vi "SEK 2019.vi"() -> ()   [LabVIEW 2016]
uses:
  <vilib>/NXT/Subs/LVHSConnector.ctl
  <vilib>/NXT/LegoClasses/BrickReference/BrickReference.lvclass
  <vilib>/NXT/Block Support/NXT_InputPort.ctl
  <vilib>/NXT/Block Support/NXT_OutputPort.ctl
  <vilib>/NXT/Dual Mode Library/Sensors/EV3_Ultrasonic_CM.vi
  <vilib>/NXT/NXTIO Xnodes/NXTIONodeSubVIs/NXTStopMotors.vi
  <vilib>/NXT/Dual Mode Library/Sensors/EV3_Color_Reflect.vi
  <vilib>/NXT/NXTIO Xnodes/NXTIONodeSubVIs/NXTMoveMotors.vi
  <vilib>/NXT/NXTIO Xnodes/AddressXNode/NXTIOAddress.xnode
  <vilib>/NXT/NXTIO Xnodes/NXTIOXNode/NXTIO.xnode
panel:
  in  "Preto EV3 (menor que y)":sgl
  in  "Branco EV3 (maior que x)":sgl=17.0
  in  "Port Ultra Topo":T1=2 items=["Port 1", "Port 2", "Port 3", "Port 4"]
  in  "Port Color Left":T1 items=["Port 1", "Port 2", "Port 3", "Port 4"]
  in  "Port Color Right":T1 items=["Port 1", "Port 2", "Port 3", "Port 4"]
  in  "Amarelo HiTechnic":i32=6
  in  "Azul HiTechnic":i32=3
  in  "Vermelho HiTechnic":i32=8
  in  "Chão (cm)":sgl=20.0
  in  "Verde HiTechnic":i32=6
  in  "Preto HiTechnic":i32
  in  "Port Gyro":T1 items=["Port 1", "Port 2", "Port 3", "Port 4"]
  in  "Port Ultra Base":T1=2 items=["Port 1", "Port 2", "Port 3", "Port 4"]
  in  "Port Color HiTechnic":T1=1 items=["Port 1", "Port 2", "Port 3", "Port 4"]
  in  "Branco HiTechnic":i32=17
  in  "NXT/EV3":T2
  # "PARÂMETROS HITECHNIC"
  # "PARÂMETROS ULTRASSOM"
  # "PORTAS DE SENSORES"
  # "PARÂMETROS COR"
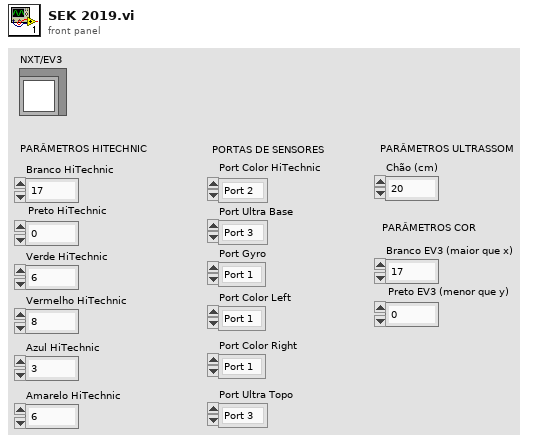
[diagram p1: front panel]
types:
  T1 = typedef "NXT_InputPort.ctl" = u32
  T2 = typedef "LVHSConnector.ctl" = refnum<class "BrickReference.lvclass">
  T3 = cluster{"Color Number":i32, "Red":i32, "Green":i32, "Blue":i32, "White Level":i32}
  T4 = typedef "NXT_OutputPort.ctl" = u8
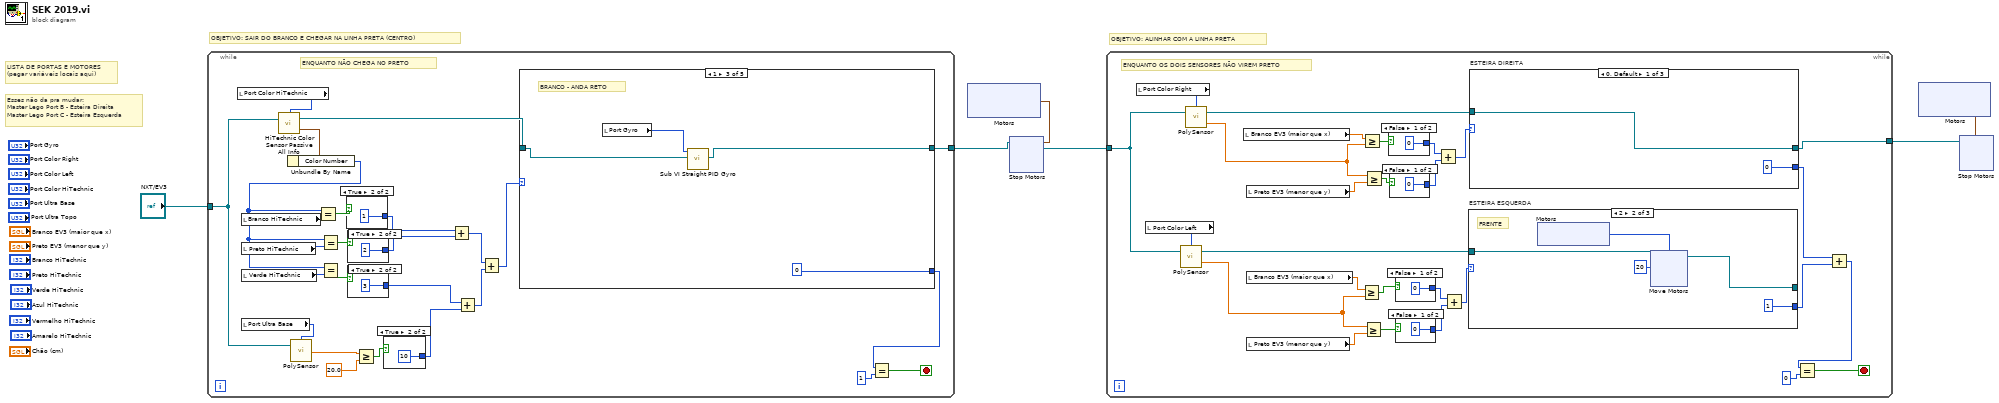
[diagram p0: block diagram]
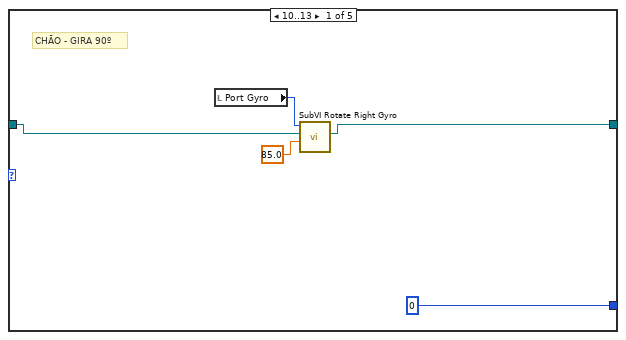
[diagram p2: hidden frame]
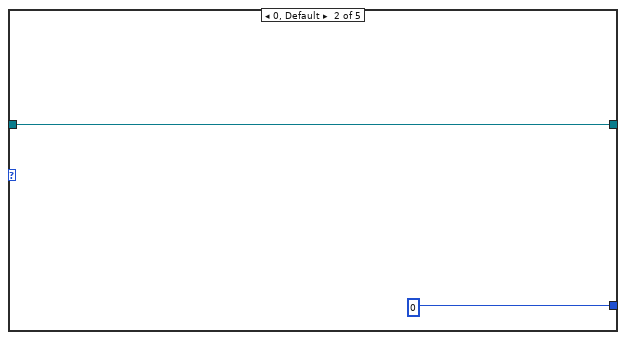
[diagram p3: hidden frame]
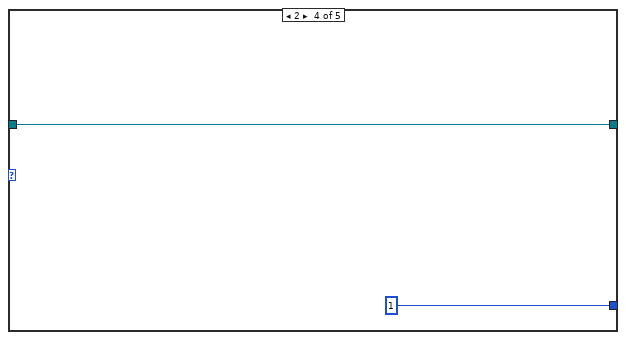
[diagram p4: hidden frame]
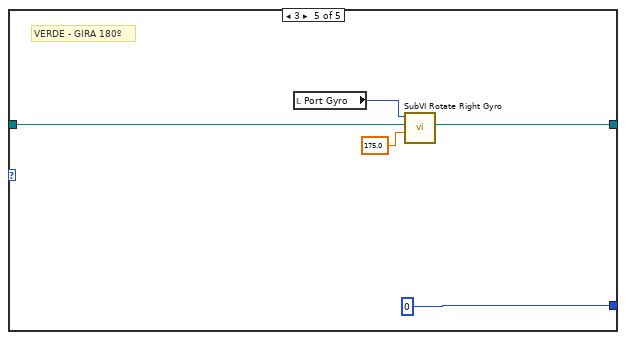
[diagram p5: hidden frame]
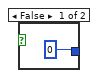
[diagram p6: hidden frame]
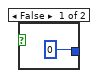
[diagram p7: hidden frame]
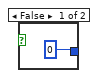
[diagram p8: hidden frame]
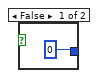
[diagram p9: hidden frame]
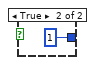
[diagram p10: hidden frame]
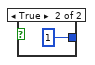
[diagram p11: hidden frame]
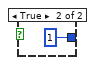
[diagram p12: hidden frame]
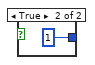
[diagram p13: hidden frame]
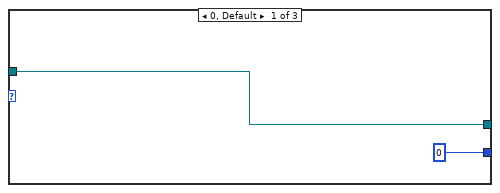
[diagram p14: hidden frame]
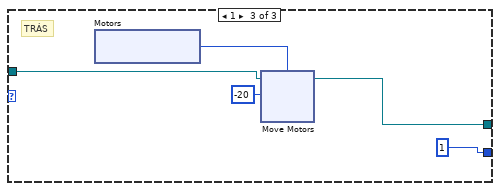
[diagram p15: hidden frame]
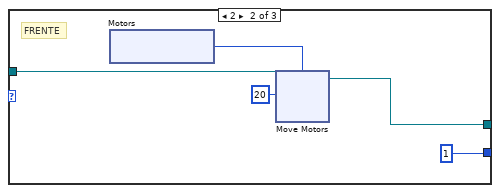
[diagram p16: hidden frame]
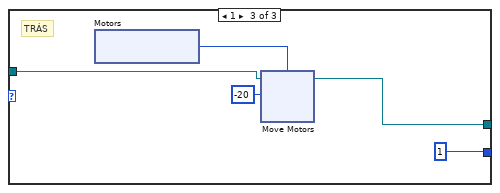
[diagram p17: hidden frame]
diagram:
  # "OBJETIVO: ALINHAR COM A LINHA PRETA"
  # "LISTA DE PORTAS E MOTORES\n(pegar variáveis locais aqui)"
  # "Esses não da pra mudar:\nMaster Lego Port B - Esteira Direita\nMaster Lego Port C - Esteira Esquerda"
  # "OBJETIVO: SAIR DO BRANCO E CHEGAR NA LINHA PRETA (CENTRO)"
  n1 = while {
    tunnel: "NXT/EV3" -> [w12]
    tunnel: [w7] -> w1
    stop <- w27 stop-if-true
    # "ENQUANTO NÃO CHEGA NO PRETO"
    n2 = local read "Port Color HiTechnic"() -> (w14:T1)
    n3 = local read "Branco HiTechnic"() -> (w25:i32)
    n4 = local read "Port Ultra Base"() -> (w9:T1)
    n5 = local read "Preto HiTechnic"() -> (w8:i32)
    n6 = local read "Verde HiTechnic"() -> (w26:i32)
    n7 = call <vilib>:"HiTechnic Color Sensor Passive All Info.vi"("NXT"=w12, "Port"=w14) -> ("All Info"=w11:T3, "NXT"=w13:T2)  [unwired: 1 in]
    n8 = Unbundle By Name(w11) -> ("Color Number"=w10:i32)
    n9 = call-poly <vilib>:"PolySensor.vi"("NXT/EV3"=w12, "Port (Port 1)"=w9) -> ("Centimeters"=w16:sgl)  [unwired: 1 in, 1 out]
    n10 = Equal?(x=w10, y=w25) -> (x = y?=w32:bool)
    n11 = Equal?(x=w10, y=w8) -> (x = y?=w31:bool)
    n12 = Equal?(x=w10, y=w26) -> (x = y?=w30:bool)
    n13 = case shown="True" w32 {
      tunnel: [0 1] -> w24
      frame False {
      }
      frame True {
      }
    }
    n14 = case shown="True" w31 {
      tunnel: [0 2] -> w23
      frame False {
      }
      frame True {
      }
    }
    n15 = case shown="True" w30 {
      tunnel: [0 3] -> w22
      frame False {
      }
      frame True {
      }
    }
    n16 = Greater Or Equal?(x=w16, y=sgl 20.0) -> (x >= y?=w17:bool)
    n17 = case shown="True" w17 {
      tunnel: [0 10] -> w21
      frame False {
      }
      frame True {
      }
    }
    n18 = Add(x=w24, y=w23) -> (x+y=w20:i32)
    n19 = Add(x=w22, y=w21) -> (x+y=w19:i32)
    n20 = Add(x=w20, y=w19) -> (x+y=w18:i32)
    n21 = case shown="1" w18 {
      tunnel: w13 -> [w35 w39 w42 w44 w49]
      tunnel: [w34 w39 w41 w44 w47] -> w7
      tunnel: [0 0 0 1 0] -> w28
      frame 10..13 {
        # "CHÃO - GIRA 90º"
        n22 = local read "Port Gyro"() -> (w33:T1)
        n23 = call "SubVI Rotate Right Gyro.vi"("angle"=85.0 ("Degrees"), "NXT/EV3"=w35, "PortGyro"=w33) -> ("NXT/EV3 2"=w34:T2)  [unwired: 7 in]
      }
      frame 0, Default {
      }
      frame 1 {
        # "BRANCO - ANDA RETO"
        n24 = local read "Port Gyro"() -> (w40:T1)
        n25 = call "Sub VI Straight PID Gyro.vi"("NXT/EV3"=w42, "PortGyro"=w40) -> ("NXT/EV3 2"=w41:T2)  [unwired: 9 in]
      }
      frame 2 {
      }
      frame 3 {
        # "VERDE - GIRA 180º"
        n26 = local read "Port Gyro"() -> (w46:T1)
        n27 = call "SubVI Rotate Right Gyro.vi"("angle"=175.0 ("Degrees"), "NXT/EV3"=w49, "PortGyro"=w46) -> ("NXT/EV3 2"=w47:T2)  [unwired: 7 in]
      }
    }
    n28 = Equal?(x=w28, y=1) -> (x = y?=w27:bool)
  }
  n29 = xnode "Motors"() -> ("Motor"=w5:cluster{"Port":T4, "Port":T4})
  n30 = xnode "Stop Motors"("Motors"=w5, "NXT/EV3"=w1) -> ("NXT/EV3"=w4:T2)
  n31 = while {
    tunnel: w4 -> [w85]
    tunnel: [w64] -> w2
    stop <- w62 stop-if-true
    # "ENQUANTO OS DOIS SENSORES NÃO VIREM PRETO"
    n32 = local read "Port Color Right"() -> (w84:T1)
    n33 = local read "Port Color Left"() -> (w83:T1)
    n34 = call-poly <vilib>:"PolySensor.vi"("NXT/EV3"=w85, "Port (Port 1)"=w83) -> ("Scaled Value"=w75:sgl, "NXT/EV3"=w81:T2)  [unwired: 1 in]
    n35 = call-poly <vilib>:"PolySensor.vi"("NXT/EV3"=w85, "Port (Port 1)"=w84) -> ("Scaled Value"=w76:sgl, "NXT/EV3"=w82:T2)  [unwired: 1 in]
    n36 = local read "Branco EV3 (maior que x)"() -> (w80:sgl)
    n37 = local read "Preto EV3 (menor que y)"() -> (w79:sgl)
    n38 = local read "Branco EV3 (maior que x)"() -> (w78:sgl)
    n39 = local read "Preto EV3 (menor que y)"() -> (w77:sgl)
    n40 = Greater Or Equal?(x=w78, y=w75) -> (x >= y?=w67:bool)
    n41 = Greater Or Equal?(x=w80, y=w76) -> (x >= y?=w74:bool)
    n42 = Greater Or Equal?(x=w75, y=w77) -> (x >= y?=w66:bool)
    n43 = Greater Or Equal?(x=w76, y=w79) -> (x >= y?=w73:bool)
    n44 = case shown="False" w74 {
      tunnel: [0 1] -> w71
      frame False {
      }
      frame True {
      }
    }
    n45 = case shown="False" w73 {
      tunnel: [0 1] -> w70
      frame False {
      }
      frame True {
      }
    }
    n46 = case shown="False" w67 {
      tunnel: [0 1] -> w69
      frame False {
      }
      frame True {
      }
    }
    n47 = case shown="False" w66 {
      tunnel: [0 1] -> w68
      frame False {
      }
      frame True {
      }
    }
    n48 = Add(x=w71, y=w70) -> (x+y=w72:i32)
    n49 = Add(x=w69, y=w68) -> (x+y=w65:i32)
    n50 = case "ESTEIRA ESQUERDA" shown="2" w65 {
      tunnel: w81 -> [w95 w99 w110]
      tunnel: [w95 w97 w111] -> _
      tunnel: [0 1 1] -> w60
      frame 0, Default {
      }
      frame 2 {
        # "FRENTE"
        n51 = xnode "Motors"() -> ("Motor"=w100:T4)
        n52 = xnode "Move Motors"("Power/Speed 1"=i8 20, "Motors"=w100, "NXT/EV3"=w99) -> ("NXT/EV3"=w97:T2)
      }
      frame 1 {
        # "TRÁS"
        n53 = xnode "Motors"() -> ("Motor"=w113:T4)
        n54 = xnode "Move Motors"("Power/Speed 1"=i8 -20, "Motors"=w113, "NXT/EV3"=w110) -> ("NXT/EV3"=w111:T2)
      }
    }
    n55 = case "ESTEIRA DIREITA" shown="0, Default" w72 {
      tunnel: w82 -> [w123 w127 w138]
      tunnel: [w123 w125 w139] -> w64
      tunnel: [0 1 1] -> w61
      frame 0, Default {
      }
      frame 2 {
        # "FRENTE"
        n56 = xnode "Motors"() -> ("Motor"=w128:T4)
        n57 = xnode "Move Motors"("Power/Speed 1"=i8 20, "Motors"=w128, "NXT/EV3"=w127) -> ("NXT/EV3"=w125:T2)
      }
      frame 1 {
        # "TRÁS"
        n58 = xnode "Motors"() -> ("Motor"=w141:T4)
        n59 = xnode "Move Motors"("Power/Speed 1"=i8 -20, "Motors"=w141, "NXT/EV3"=w138) -> ("NXT/EV3"=w139:T2)
      }
    }
    n60 = Add(x=w61, y=w60) -> (x+y=w59:i32)
    n61 = Equal?(x=w59, y=0) -> (x = y?=w62:bool)
  }
  n62 = xnode "Motors"() -> ("Motor"=w3:cluster{"Port":T4, "Port":T4})
  n63 = xnode "Stop Motors"("Motors"=w3, "NXT/EV3"=w2) -> ()  [unwired: 1 out]
